vi "Write ADU Packet Slave.vi"(7 "Slave (F)":bool, 8 "error in (no error) 2":errorcluster, 9 "Modbus Data Unit":T2={"Function Code"=enum."Read Coils", "Data"=[]} {"Data" format="%.0x"}, 10 "MBAP Header":T1, 11 "TCP in":refnum<class "TCP.lvclass">) -> (0 "error out 2":errorcluster, 2 "Transaction ID RD":u16, 3 "TCP out":refnum<class "TCP.lvclass">)   [LabVIEW 2019]
doc: "This uses the protocol layer to write a modbus packet to the bus, wrapped in the IP transmission data unit."
uses:
  Ctl/MB Modbus Data Unit.ctl
  TCP/TCP.lvclass
  TCP/TCP.lvclass/TCP.ctl
  NI_modbus_upd.lvlib
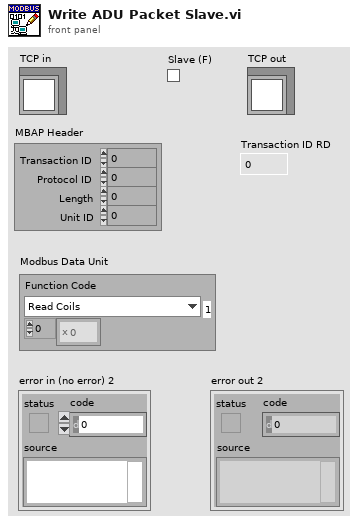
[diagram p1: front panel]
types:
  T1 = cluster{"Transaction ID":u16, "Protocol ID":u16, "Length":u16, "Unit ID":u8}
  T2 = typedef "NI_modbus_upd.lvlib/MB Modbus Data Unit.ctl" = cluster{"Function Code":enum16{"Read Discrete Inputs", "Read Coils", "Write Single Coil", "Write Multiple Coils", "Read Input Register", "Read Holding Registers", "Write Single Register", "Write Multiple Registers", "Read/Write Multiple Registers", "Mask Write Register", "Read FIFO Queue", "Read File Record", "Write File Record", "Read Exception Status", "Diagnostic", "Get Com Event Counter", "Get Com Event Log", "Report Slave ID", "Read Device Identification"}, "Data":u8[]}
  T3 = enum16{"Read Discrete Inputs", "Read Coils", "Write Single Coil", "Write Multiple Coils", "Read Input Register", "Read Holding Registers", "Write Single Register", "Write Multiple Registers", "Read/Write Multiple Registers", "Mask Write Register", "Read FIFO Queue", "Read File Record", "Write File Record", "Read Exception Status", "Diagnostic", "Get Com Event Counter", "Get Com Event Log", "Report Slave ID", "Read Device Identification"}
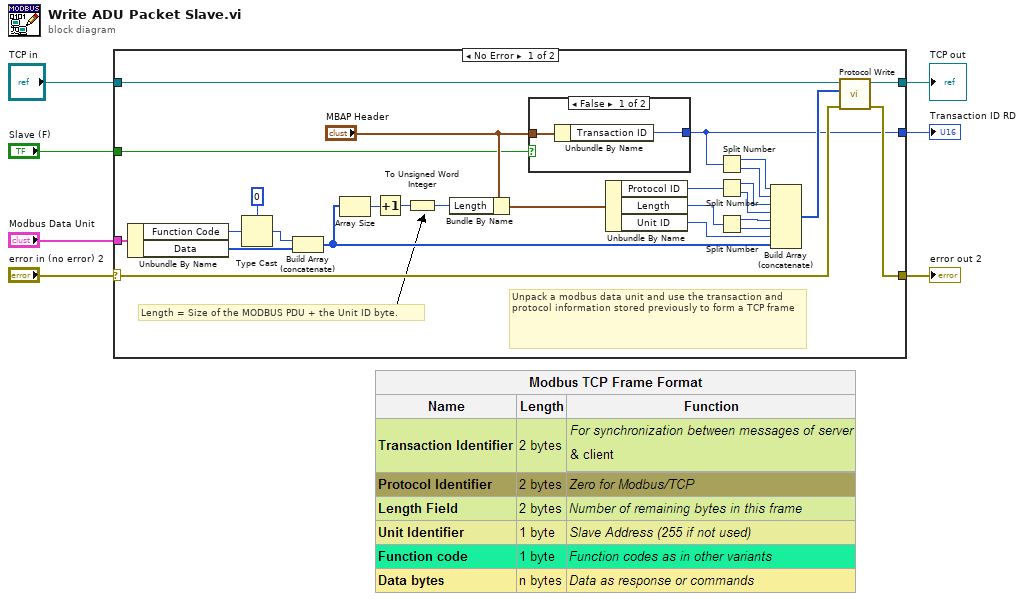
[diagram p0: block diagram]
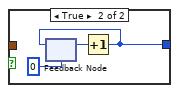
[diagram p2: hidden frame]
diagram:
  n1 = case shown="No Error" "error in (no error) 2" {
    selector: "error in (no error) 2" -> [w12 w41]
    tunnel: "Modbus Data Unit" -> [w34 _]
    tunnel: "TCP in" -> [w14 w40]
    tunnel: [w13 w40] -> w5
    tunnel: [w11 w41] -> w3
    tunnel: "Slave (F)" -> [w9 _]
    tunnel: [w8 _] -> w1
    frame No Error {
      # "Unpack a modbus data unit and use the transaction and protocol information stored previously to form a TCP frame"
      # "Length = Size of the MODBUS PDU + the Unit ID byte."
      n2 = Unbundle By Name(w34) -> ("Function Code"=w31:T3, "Data"=w30:u8[])
      n3 = Type Cast(type=u8 0, x=w31) -> (*(type *) &x=w33:u8)
      n4 = Build Array (concatenate)(w33, w30) -> (w18:u8[])
      n5 = Array Size(array=w18) -> (size(s)=w22:i32)
      n6 = Increment(x=w22) -> (x+1=w21:i32)
      n7 = To Unsigned Word Integer(number=w21) -> (unsigned 16bit integer=w20:u16)
      n8 = Bundle By Name(cluster="MBAP Header", "Length"=w20) -> (w19:T1)
      n9 = case shown="False" w9 {
        tunnel: "MBAP Header" -> [w35 _]
        tunnel: [w36 w37] -> w8
        frame False {
          n10 = Unbundle By Name(w35) -> ("Transaction ID"=w36:u16)
        }
        frame True {
          n11 = feedback #1(u16 0) -> (w38:u16)
          n12 = Increment(x=w38) -> (x+1=w37:u16)
          n13 = feedback-in #1(w37) -> ()
        }
      }
      n14 = Unbundle By Name(w19) -> ("Protocol ID"=w29:u16, "Length"=w16:u16, "Unit ID"=w17:u8)
      n15 = Split Number(x=w8) -> (hi(x)=w28:u8, lo(x)=w27:u8)
      n16 = Split Number(x=w29) -> (hi(x)=w26:u8, lo(x)=w25:u8)
      n17 = Split Number(x=w16) -> (hi(x)=w24:u8, lo(x)=w23:u8)
      n18 = Build Array (concatenate)(w28, w27, w26, w25, w24, w23, w17, w18) -> (w15:u8[])
      n19 = call "Protocol Write.vi"("error in (no error)"=w12, "data"=w15, "protocol layer in"=w14) -> ("error out"=w11:errorcluster, "protocol layer out"=w13:refnum<class "TCP.lvclass">)  [unwired: 6 in, 1 out]
    }
    frame Error {
    }
  }
  "TCP out" <- w5
  "error out 2" <- w3
  "Transaction ID RD" <- w1
